vi "Add Subsystem Reference.vi"(8 "error in (no error)":errorcluster, 10 "LabVIEW Object":refnum<class>, 11 "TopLevel in":refnum<class "Motor Controller.lvclass">) -> (0 "error out":errorcluster, 3 "TopLevel out":refnum<class "Motor Controller.lvclass">)   [LabVIEW 2022 SP3, in "Motor Controller.lvclass"]
uses:
  Motor Controller.lvclass
  Motor Controller.lvclass/Motor Controller.ctl
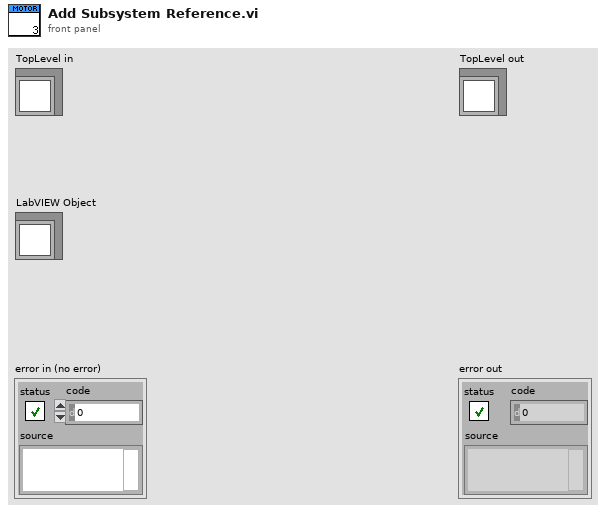
[diagram p1: front panel]
types:
  T1 = typedef "Motor Controller.lvclass/Private Data.ctl" = cluster{"UserEvents":T2, "All Dependencies":cluster{"Class References":refnum<class>[], "Class Names":string[]}, "Status":T3}
  T2 = typedef "Motor Controller.lvclass/UserEvents.ctl" = cluster{"API Incoming Event":refnum<user-event>, "API Executed Event":refnum<user-event>, "API Return Event":refnum<user-event>, "Status Changed Event":refnum<user-event>, "StopEvent":refnum<user-event>}
  T3 = typedef "Motor Controller.lvclass/Status.ctl" = cluster{"Motor Controller Config Data":T4, "Motor Controller Data":cluster{"Enabled?":bool}, "Stage Move":T5, "Stage Busy?":bool}
  T4 = typedef "Motor Controller.lvclass/Motor Controller Config Data.ctl" = cluster{"Motor IP Addresss":string, "Current Position":i32, "Pulse_Per_mm":i32, "PrePrint":dbl[], "Load Position_mm":i32, "Laminate Position_mm":i32}
  T5 = typedef "Motor Controller.lvclass/Stage Move Data.ctl" = cluster{"Current Step":string, "Move Data":T6[]}
  T6 = typedef "Motor Controller.lvclass/Batch Index Speed Data.ctl" = cluster{"Batch & Cycle":string, "Move":cluster{"Index_mm":i32, "Speed_mm_s":i32}, "Status":T7}
  T7 = typedef "Motor Controller.lvclass/Move Status.ctl" = enum16{"Pending", "In Progress", "Completed"}
  T8 = cluster{"Class References":refnum<class>[], "Class Names":string[]}
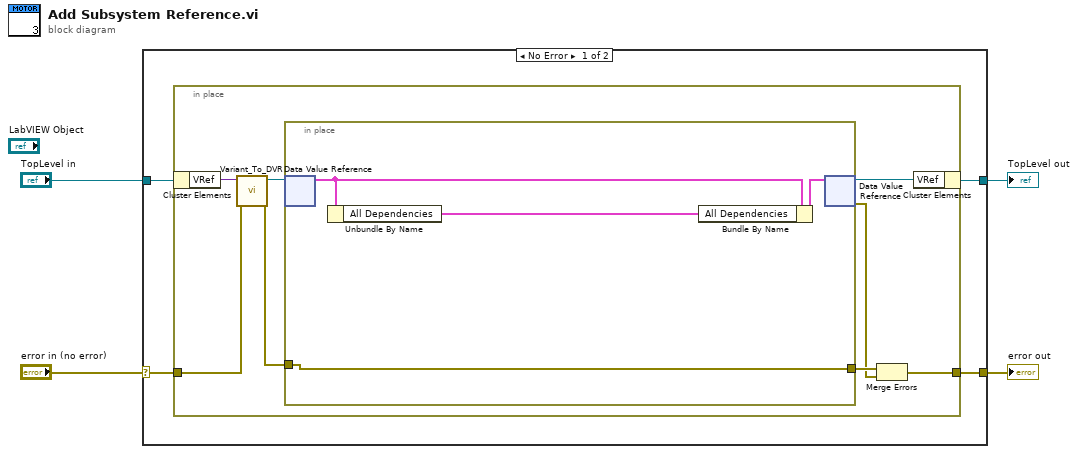
[diagram p0: block diagram]
diagram:
  n1 = case shown="No Error" "error in (no error)" {
    selector: "error in (no error)" -> [w5 w22]
    tunnel: [w7 w22] -> w3
    tunnel: [w8 w21] -> w1
    tunnel: "TopLevel in" -> [w6 w21]
    frame No Error {
      n2 = in-place {
        in-place-border: w5 -> [w14]
        in-place-border: [w10] -> w7
        n3 = in-place-cluster #1(w6) -> ("VRef"=w16:variant)
        n4 = call "Variant_To_DVR.vi"("error in (no error)"=w14, "Variant"=w16) -> ("error out"=w13:errorcluster, "DVR"=w15:refnum<data-value>)  [unwired: 8 in]
        n5 = in-place {
          in-place-border: w13 -> [w18]
          in-place-border: [w18] -> w12
          n6 = in-place-dvr #2(w15) -> (w20:T1)  [unwired: 1 out]
          n7 = Unbundle By Name(w20) -> ("All Dependencies"=w17:T8)
          n8 = Bundle By Name(cluster=w20, "All Dependencies"=w17) -> (w19:T1)
          n9 = in-place-dvr #2(w19) -> (w9:refnum<data-value>, w11:errorcluster)
        }
        n10 = Merge Errors(w12, w11) -> (w10:errorcluster)
        n11 = in-place-cluster #1("VRef"=w9) -> (w8:refnum<class "Motor Controller.lvclass">)
      }
    }
    frame Error {
    }
  }
  "error out" <- w3
  "TopLevel out" <- w1
